vi "ROVPingRead.vi"(8 "error in (no error)":errorcluster, 11 "VISA Refnum in":refnum<visa-resource-name>) -> (0 "error out":errorcluster, 1 "Afstand Ping1D (m)":dbl, 2 "Ping1d svar":string, 3 "VISA Refnum out":refnum<visa-resource-name>)   [LabVIEW 2021]
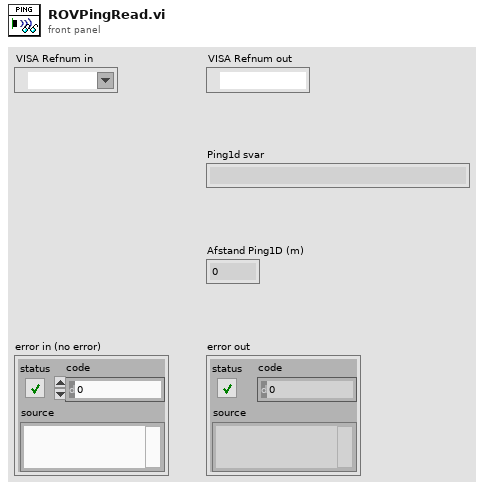
[diagram p1: front panel]
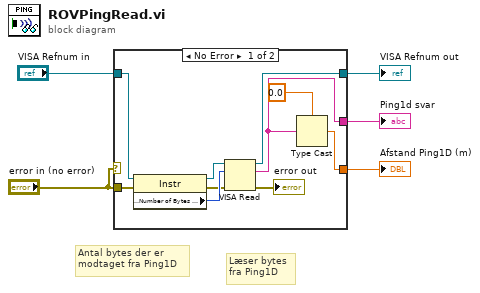
[diagram p0: block diagram]
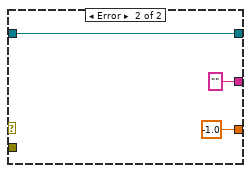
[diagram p2: hidden frame]
diagram:
  # "Læser bytes \nfra Ping1D"
  # "Antal bytes der er\nmodtaget fra Ping1D"
  n1 = case shown="No Error" "error in (no error)" {
    tunnel: [w15 -1.0 ("Afstand Ping1D (m)")] -> w5
    tunnel: [w13 w18] -> w4
    tunnel: [w11 "" ("read buffer")] -> w3
    tunnel: "VISA Refnum in" -> [w7 w18]
    tunnel: "error in (no error)" -> [w6 _]
    frame No Error {
      n2 = property class="Instr"(reference=w7, error in=w6) -> (reference out=w8:refnum<visa-resource-name>, error out=w9:errorcluster, "Serial Settings:Number of Bytes at Serial Port"=w10:u32)
      n3 = VISA Read(VISA resource name=w8, byte count=w10, error in (no error)=w9) -> (VISA resource name out=w13:refnum<visa-resource-name>, read buffer=w11:string, error out=→"error out":errorcluster)  [unwired: 1 out]
      n4 = Type Cast(type=0.0 ("Afstand Ping1D (m)"), x=w11) -> (*(type *) &x=w15:dbl)
    }
    frame Error {
    }
  }
  "Ping1d svar" <- w3
  "Afstand Ping1D (m)" <- w5
  "VISA Refnum out" <- w4
